vi "tm_startcapture_a.vi"(8 "error in (no error)":errorcluster, 9 "Frames":i32, 10 "Capture mode":i32(ring) items=["Snap", "Sequence"], 11 "Handle in":u32) -> (0 "error out":errorcluster, 2 "Buffer":u16[][](array[numeric]), 3 "Handle out":u32, 4 "Image type":u32)   [LabVIEW 2011]
uses:
  tmcamcon.dll
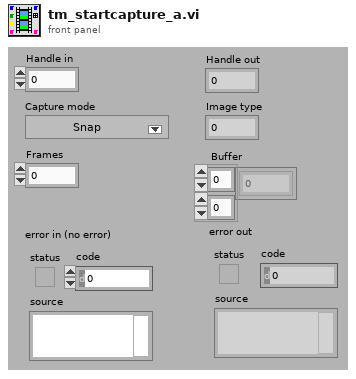
[diagram p1: front panel]
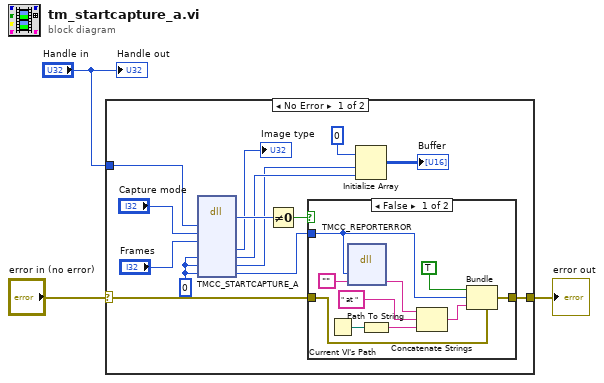
[diagram p0: block diagram]
diagram:
  n1 = case shown="No Error" "error in (no error)" {
    selector: "error in (no error)" -> [w12 w29]
    tunnel: [w11 w29] -> w1
    tunnel: "Handle in" -> [w16 _]
    frame No Error {
      w4 = 0 ("Erval")
      n2 = dll-call lib="tmcamcon.dll" fn="TMCC_STARTCAPTURE_A"("index"=w16, "mode"="Capture mode", "frames"="Frames", "width"=w4, "height"=w4, "Erval"=w4) -> ("return type"=w17:u32, "datatype"=→"Image type":u32, "width"=w6:i32, "height"=w5:i32, "Erval"=w13:i32)  [unwired: 7 in, 2 out]
      n3 = Not Equal To 0?(x=w17) -> (x != 0?=w14:bool)
      n4 = case shown="False" w14 {
        tunnel: w12 -> [w27 w28]
        tunnel: [w26 w28] -> w11
        tunnel: w13 -> [w20 _]
        frame False {
          n5 = Current VI's Path() -> (path=w25:path)
          n6 = dll-call lib="tmcamcon.dll" fn="TMCC_REPORTERROR"("error"=w20, "buf"="") -> ("buf"=w19:string)  [unwired: 5 in, 2 out]
          n7 = Path To String(path=w25) -> (string=w21:string)
          n8 = Concatenate Strings(w19, " at ", w21) -> (w24:string)
          n9 = Bundle(cluster=w27, "status"=TRUE, "code"=w20, "source"=w24) -> (w26:errorcluster)
        }
        frame True {
        }
      }
      n10 = Initialize Array(u16 0, w5, w6) -> (→"Buffer":u16[][])
    }
    frame Error {
    }
  }
  "error out" <- w1
  "Handle out" <- "Handle in"
